vi "Dashboard Main.vi"() -> ()   [LabVIEW 2015]
uses:
  <vilib>/Utility/miscctls.llb/LVRowAndColumnTypeDef.ctl
  <vilib>/event_ctls.llb/eventvkey.ctl
  <vilib>/Rock Robotics/WPI/Dashboard/WPI_DashboardLogging Global.vi
  <vilib>/Rock Robotics/Network Tables/NT Read Numeric Array.vi
  <vilib>/Utility/config.llb/Write Key (String).vi
  <vilib>/Utility/config.llb/Write Key (I32).vi
  <vilib>/Utility/config.llb/NI_LVConfig.lvlib
  <vilib>/vision/NI_Vision_Development_Module.lvlib
panel:
  out "fps 2":dbl format="%#.1g"
  in  "Camera Settings 2":T1={"Frame Rate"=30, "Compression"=30, "Size"=1} {"Frame Rate" scale=1.0..30.0; "Size" items=["640x480", "320x240", "160x120"]}
  in  "Vision 2":u16(ring) items=["Camera Off", "USB Camera SW", "USB Camera HW", "IP Camera"]
  out "Mbps 2":dbl format="%#.1g"
  in  "TCP":refnum<k5>
  in  "Rec Mode":enum32{"Stop", "Record", "Playback"}(radio)
  in  "Vision":u16(ring) items=["Camera Off", "USB Camera SW", "USB Camera HW", "IP Camera"]
  out "Camera IP":string
  out "Image Message":string="Timeout in Camera Communications"
  in  "Dashboard Tab":T2(tab)
  in  "Select Auto":string(combo)
  out "NT Connection":bool
  in  "Camera Settings":T1={"Frame Rate"=30, "Compression"=30, "Size"=1} {"Frame Rate" scale=1.0..30.0; "Size" items=["640x480", "320x240", "160x120"]}
  out "MotorChart R":cluster{"Numeric":dbl, "Numeric":dbl}(graph)
  out "MotorChart L":T3(graph)
  out "MotorSliders R":cluster{"MotorSlide1":dbl, "MotorSlide2":dbl} {"MotorSlide2" scale=-1.0..1.0 scale format="%#_2e"; "MotorSlide1" scale=-1.0..1.0 scale format="%#_2e"}
  out "MotorSliders L":T4 {"MotorSlide4 2" scale=0.0..14.0 scale format="%#_2e"; "MotorSlide2" scale=-1.0..1.0 scale format="%#_2e"; "MotorSlide1" scale=-1.0..1.0 scale format="%#_2e"}
  out "Gyro":dbl(knob) scale=0.0..360.0
  out "JS1 Z":dbl(slide) scale=-1.0..1.0 scale format="%#_2e"
  out "JS1 Graph":cluster{"X":dbl, "Y":dbl}[](graph)
  out "JS1 Buttons":T5
  out "JS2 Z":dbl(slide) scale=-1.0..1.0 scale format="%#_2e"
  out "JS2 Graph":cluster{"X":dbl, "Y":dbl}[](graph)
  out "JS2 Buttons":T5
  out "Mode":T6(ring)=enum."Auto Disabled"
  in  "DB Camera Config":bool
  out "fps":dbl format="%#.1g"
  out "Mbps":dbl format="%#.1g"
  out "Mbps LED":bool
  in  "DB/String 9":string
  in  "DB/String 8":string
  in  "DB/String 7":string
  in  "DB/String 6":string
  in  "DB/String 5":string
  in  "DB/String 4":string
  in  "DB/String 3":string
  in  "DB/String 2":string
  in  "DB/String 1":string
  in  "DB/String 0":string
  in  "DB/Slider 0":dbl(slide) scale=0.0..5.0
  in  "DB/Slider 1":dbl(slide) scale=0.0..5.0
  in  "DB/Slider 2":dbl(slide) scale=0.0..5.0
  in  "DB/Slider 3":dbl(slide) scale=0.0..5.0
  out "DB/LED 3":bool
  out "DB/LED 2":bool
  out "DB/LED 1":bool
  out "DB/LED 0":bool
  in  "DB/Button 3":bool
  in  "DB/Button 2":bool
  in  "DB/Button 1":bool
  in  "DB/Button 0":bool caption="New Name"
  in  "Test Slider":dbl(slide) scale=0.0..100.0 scale format="%#_3g"
  in  "On/Off":bool caption="Solenoid"
  in  "Test Name":u16(ring) items=["Select the test to run..."]
  in  "Test Tree":string(tree)
  in  "Motor":cluster{"Value":dbl, "Enable":bool} {"Value" scale=-1.0..1.0 scale format="%#_3g"}
  out "Progress":T7 {"Test Progress" scale=0.0..100.0}
  in  "Rev/Fwd":cluster{"Forward":bool, "Reverse":bool}
  in  "Test Ring":u16(ring) items=["Monochrome", "Color"]
  out "Cmd Status":string
  in  "Execute Command":bool
  in  "Command Params":string[][](table)
  in  "Command Selection":i32(listbox)
  in  "CheckList":i32(listbox)
  out "Tree":string(tree)
  out "Camera Image":T8(plugin-control)
  out "Background":bool
  # "Left"
  # "Front"
  # "Right"
  # "Battery"
  # "This tab is a great place for autonomous settings and robot-specific values.\nPlace controls and indicators inside this tab and match name to\nDashboard Variables on robot. You can also delete this comment."
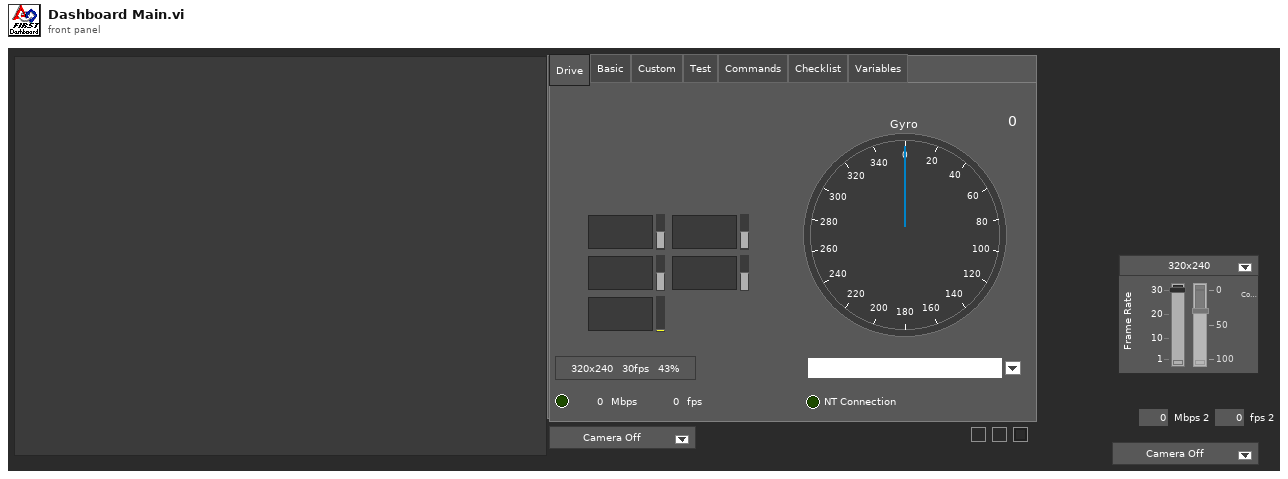
[diagram p1: front panel]
types:
  T1 = cluster{"Frame Rate":i32, "Compression":i32, "Size":u16}
  T2 = enum32{"Drive", "Basic", "Custom", "Test", "Commands", "Checklist", "Variables"}
  T3 = cluster{"Numeric":dbl, "Numeric":dbl, "Battery V":dbl}
  T4 = cluster{"MotorSlide1":dbl, "MotorSlide2":dbl, "MotorSlide4 2":dbl}
  T5 = cluster{bool, bool, bool, bool, bool, bool, bool, bool, bool, bool, bool, bool}
  T6 = enum8{"Tele-Op Disabled", "Tele-Op Enabled", "Auto Disabled", "Auto Enabled", "Test Disabled", "Test Enabled", "Disconnected", "No Code", "E-Stop"}
  T7 = cluster{"Test Progress":u8, "Test Progress Text":string}
  T8 = typedef "IMAQ Image.ctl" = refnum<image>
  T9 = typedef "Image Type" = u32
  T10 = cluster{"IDs":cluster{"RPC field ID":u16, "Unique ID":u16}, "String":string}
  T11 = enum32{"Drive", "Basic", "Custom", "Test", "Checklist", "Variables"}
  T12 = cluster{"Camera Image":refnum<vi>, "Dashboard Tab":refnum<vi>, "Background":refnum<vi>, "Vision":refnum<vi>, "Rec Mode":refnum<vi>, "Test Slider":refnum<vi>, "On/Off ":refnum<vi>, "Test Ring":refnum<vi>, "Rev/Fwd":refnum<vi>, "Test Name":refnum<vi>, "Motor":refnum<vi>, "Progress":refnum<vi>, "CheckList":refnum<vi>, "Tree":refnum<vi>, "Test Tree":refnum<vi>, "Command Params":refnum<vi>, "Command Selection":refnum<vi>, "Execute Command":refnum<vi>, "Cmd Status":refnum<vi>}
  T13 = cluster{"Error Strings":string, "Disable Counts":cluster{u16, u16}, "Rail Faults":cluster{u16, u16, u16}, "Robot IP":string, "DB Mode":u8, "Event Info":cluster{"Name":string, "Type":u8, "Number":u16, "Replay":u8}, "Camera Addr":string}
  T14 = cluster{"Storage":cluster{"Disk Free":u64, "RAM Block":u32, "RAM free":u32}, "CPU Utilization":cluster{"CPU % ISR":sgl, "CPU % Time Crit":sgl, "CPU % Timed Str":sgl, "CPU % High":sgl, "CPU % Above":sgl, "CPU % Normal":sgl, "CPU % Low":sgl}, "CAN":cluster{"% Bus Utilization":sgl, "Bus Off Cnt":u32, "TX_FIFO Full Cnt":u32, "Receive Error Cnt":u8, "Transmit Error Cnt":u8}, "HID":cluster{"HID Outputs":u32, "Rumble Low":u16, "Rumble High":u16}[]}
  T15 = cluster{"Status bits":cluster{"Test Mode":bool, "Autonomous":bool, "Enabled":bool, "Code Start":bool, "Brownout":bool, "Reserved 2":bool, "Reserved 3":bool, "E-Stop":bool}, "Code Trace":cluster{"Disabled":bool, "TeleOp":bool, "Auto":bool, "Test":bool}, "Controller Type":enum16{"unknown", "cRIO", "roboRio"}, "Code?":enum16{"unknown", "noCode", "code"}, "Battery V":dbl}
  T16 = cluster{"Control Bits":cluster{"TestMode":bool, "Autonomous":bool, "Enabled":bool, "FMS Present":bool, bool, bool, bool, "E-Stop":bool}, "Team Station ":u8, "Countdown":sgl, "Joystick Values":cluster{"Axes":dbl[], "Buttons":bool[], "POVs":i16[]}[]}
  T17 = cluster{"Axes":dbl[], "Buttons":bool[], "POVs":i16[]}[]
  T18 = cluster{"Axes":dbl[], "Buttons":bool[], "POVs":i16[]}
  T19 = cluster{"Buttons[0]":bool, "Buttons[1]":bool, "Buttons[2]":bool, "Buttons[3]":bool, "Buttons[4]":bool, "Buttons[5]":bool, "Buttons[6]":bool, "Buttons[7]":bool, "Buttons[8]":bool, "Buttons[9]":bool, "Buttons[10]":bool, "Buttons[11]":bool}
  T20 = typedef "NI_LVConfig.lvlib/Config Data RefNum.ctl" = refnum<k1>
  T21 = cluster{"Operation":enum16{"Update", "Clear"}, "Color Box":u32}[]
  T22 = typedef "eventvkey.ctl" = enum16{"ASCII", "Enter", "Return", "Shift", "Ctrl", "Alt", "Cmd", "Opt", "Caps", "NumLock", "Clear", "Break", "Up", "Down", "Left", "Right", "Insert", "Delete", "Home", "End", "PageUp", "PageDown", "Escape", "Help", "Pause", "ScrollLock", "F1", "F2", "F3", "F4", "F5", "F6", "F7", "F8", "F9", "F10", "F11", "F12", "F13", "F14", "F15", "F16", "F17", "F18", "F19", "F20", "F21", "F22", "F23", "F24", "Play", "VolumeUp", "VolumeDown", "Mute", "Two Byte Char"}
  T23 = cluster{"Image Size":bool, "Image Type":bool, "Pixel Value":bool, "ROI Information":bool, "Zoom Factor":bool}
  T24 = enum8{"Enabled", "Disabled", "Disabled and Grayed Out"}
  T25 = cluster{"Operation":enum16{"Update", "Clear"}, "Color Box":u32}
  T26 = typedef "LVRowAndColumnTypeDef.ctl" = cluster{"Row":i32, "Column":i32}
  T27 = cluster{"Shift":bool, "Ctrl":bool, "Alt":bool, "Cmd":bool, "Opt":bool}
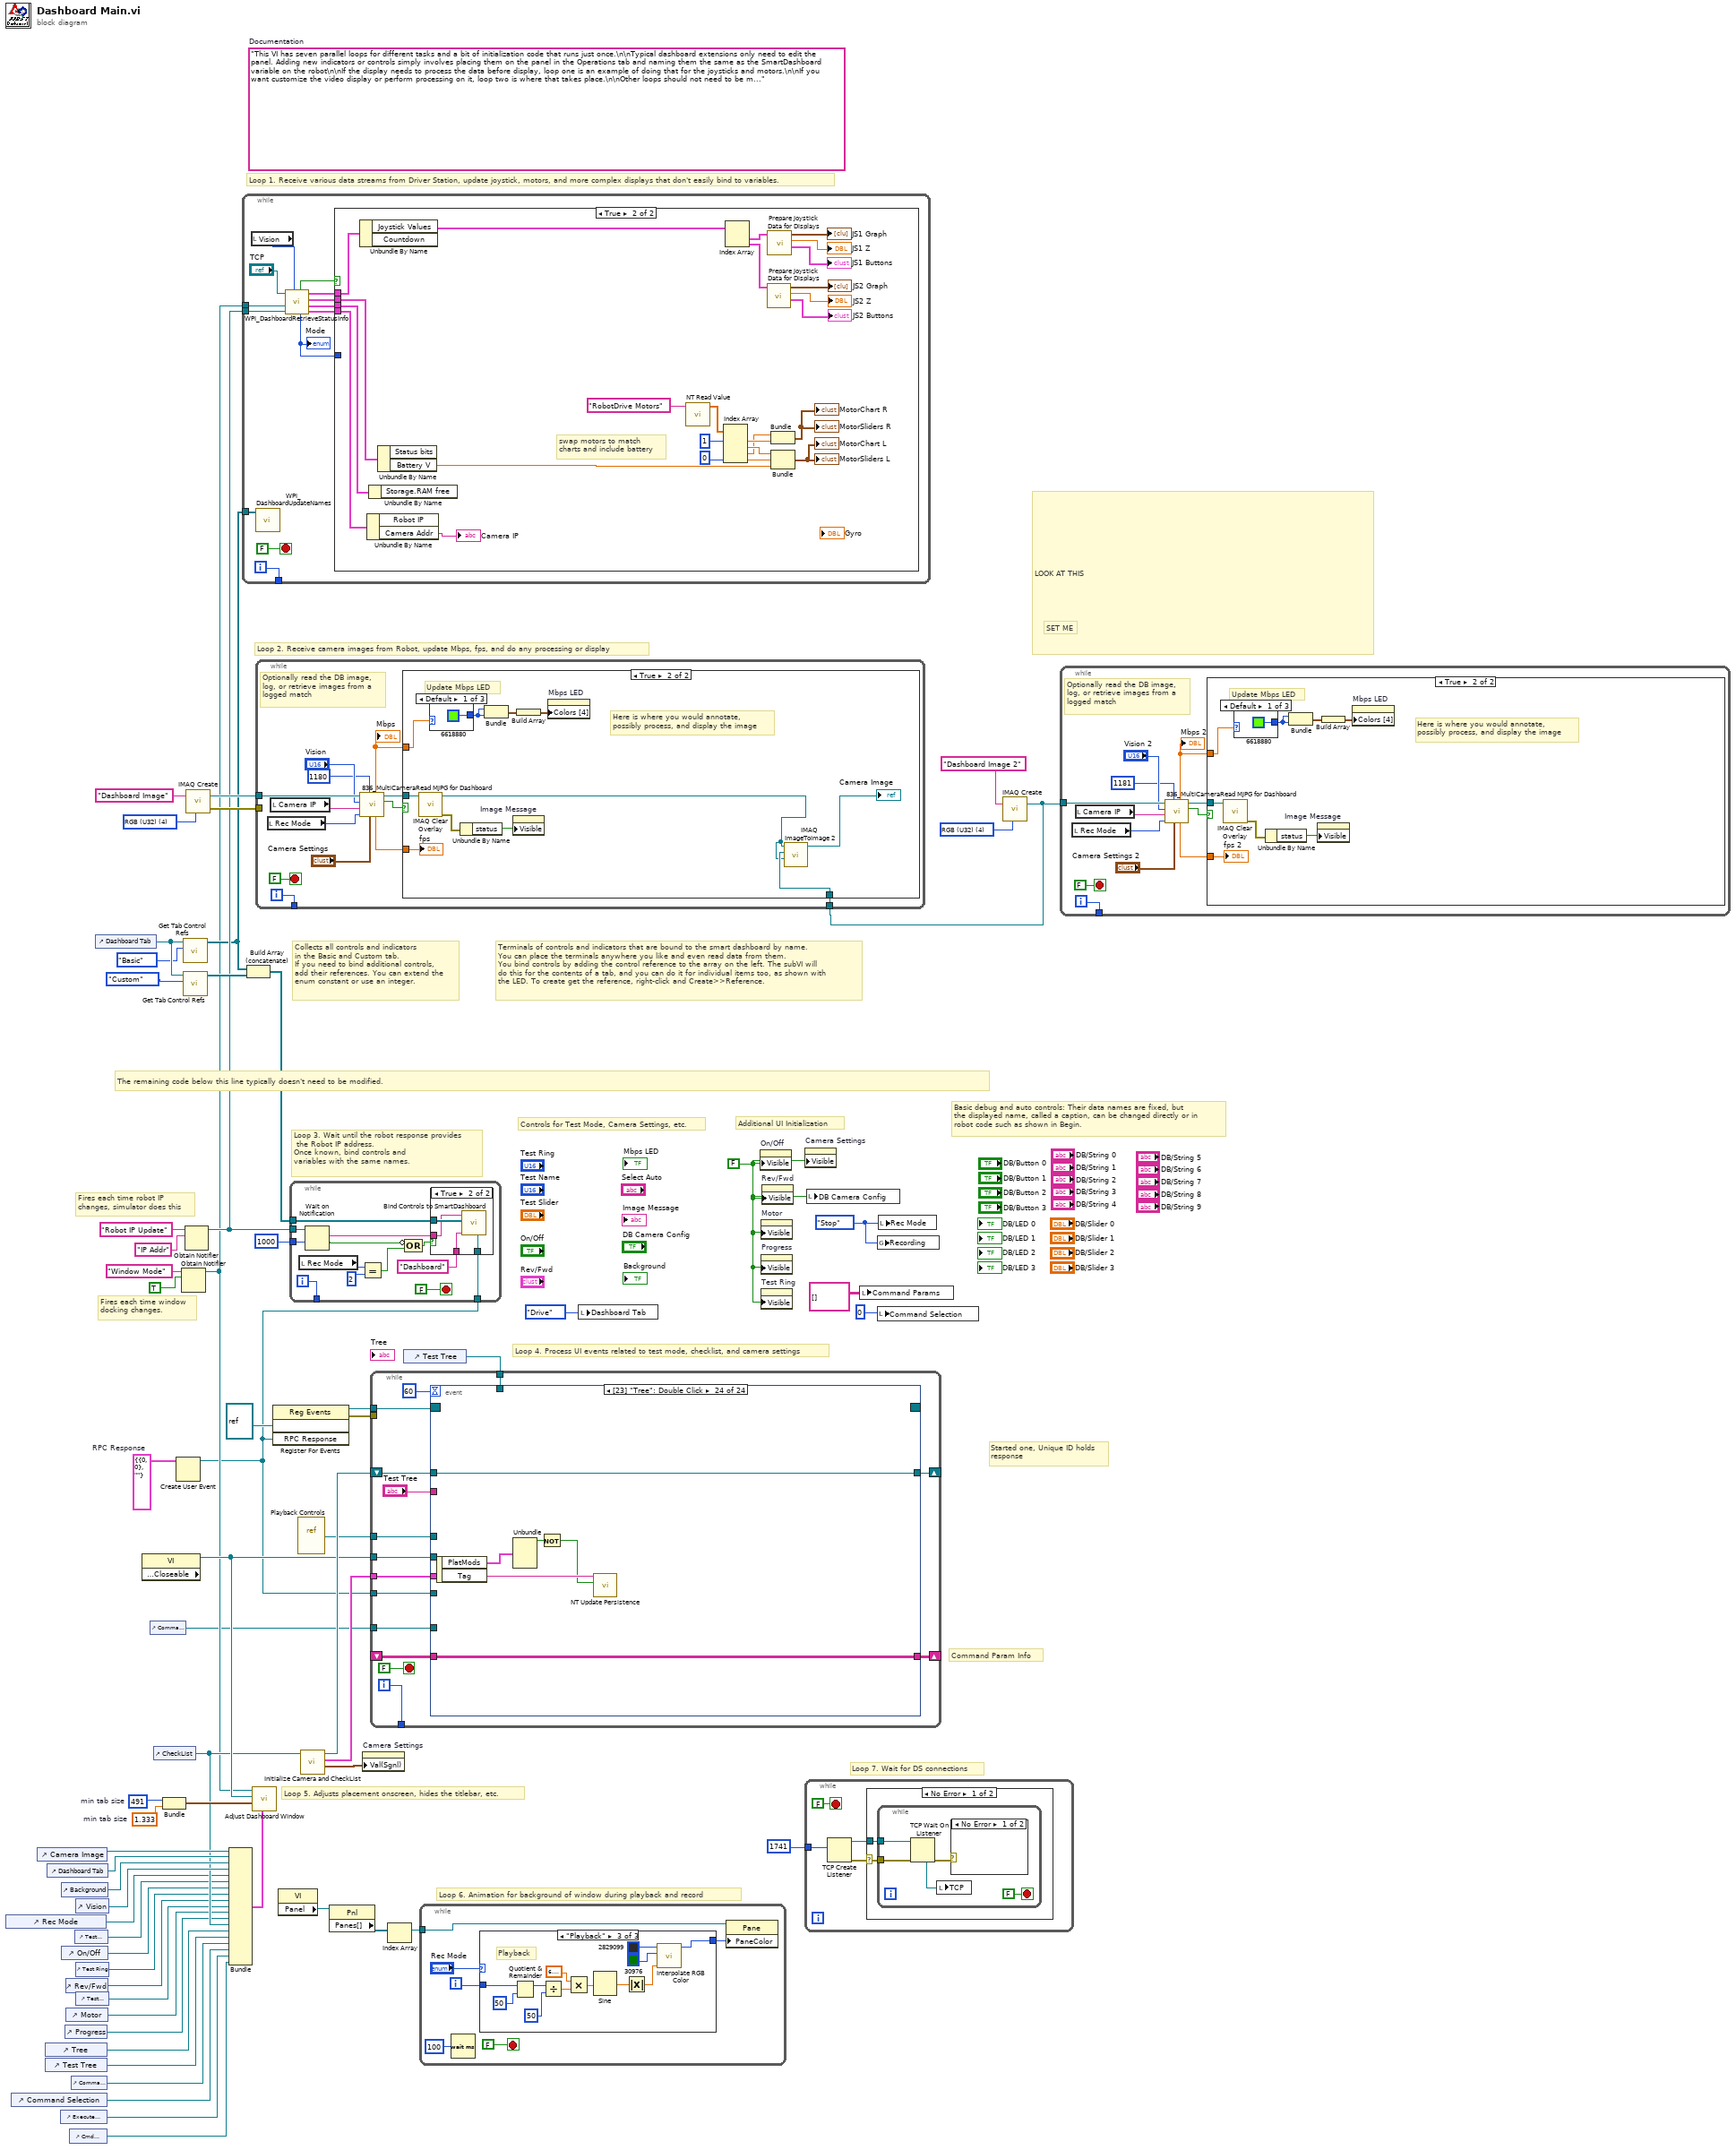
[diagram p0: block diagram]
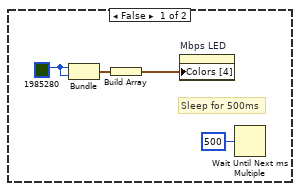
[diagram p2: hidden frame]
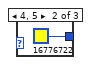
[diagram p3: hidden frame]
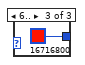
[diagram p4: hidden frame]
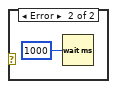
[diagram p5: hidden frame]
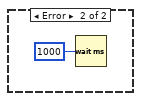
[diagram p6: hidden frame]
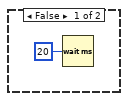
[diagram p7: hidden frame]
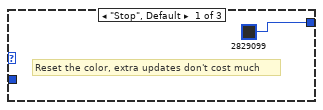
[diagram p8: hidden frame]
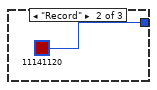
[diagram p9: hidden frame]
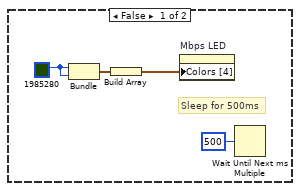
[diagram p11: hidden frame]
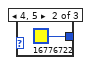
[diagram p12: hidden frame]
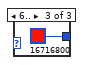
[diagram p13: hidden frame]
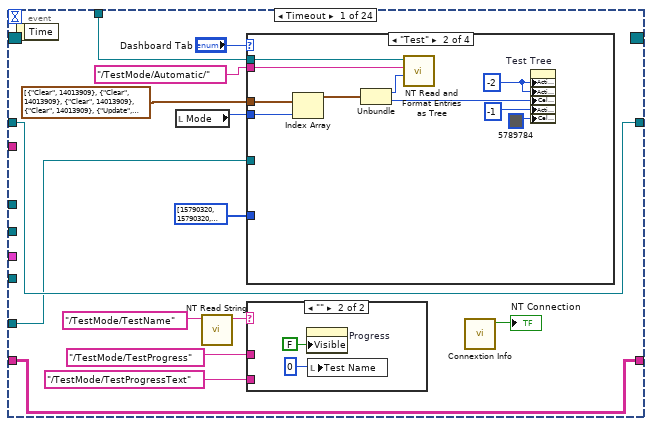
[diagram p14: hidden frame]
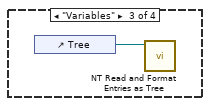
[diagram p16: hidden frame]
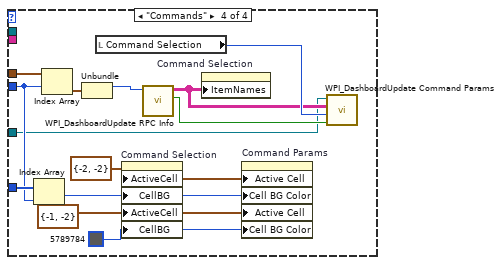
[diagram p17: hidden frame]
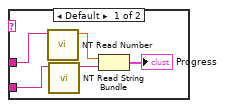
[diagram p18: hidden frame]
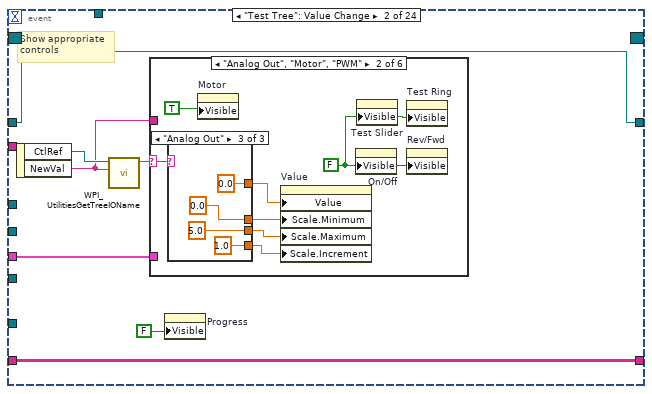
[diagram p19: hidden frame]
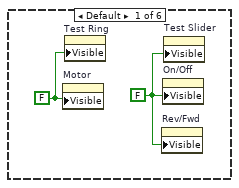
[diagram p20: hidden frame]
diagram:
  w2 = T9 4 items=["Grayscale (U8)", "Grayscale (I16)", "Grayscale (SGL)", "Complex (CSG)", "RGB (U32)", "HSL (U32)", "RGB (U64)"] ("Image Type")
  w10 = T10 {"IDs"={"RPC field ID"=0, "Unique ID"=0}, "String"=""}  # RPC Response
  w36 = 491  # min tab size
  w35 = 1.333  # min tab size
  w44 = enum32{"Stop", "Record", "Playback"}."Stop" ("Rec Mode")
  w18 = FALSE ("Visible")
  (unwired) "This VI has seven parallel loops for different tasks and a bit of initialization code that runs just once.\n\nTypical dashboard extensions only need to edit the panel. Adding new indicators or controls simply involves placing them on the panel in the Operations tab and naming them the same as the SmartDashboard variable on the robot\n\nIf the display needs to process the data before display, loop one is an example of doing that for the joysticks and motors.\n\nIf you want customize the video display or perform processing on it, loop two is where that takes place.\n\nOther loops should not need to be modified. They are pretty standard, and document the task they perform."  # Documentation
  w64 = T9 4 items=["Grayscale (U8)", "Grayscale (I16)", "Grayscale (SGL)", "Complex (CSG)", "RGB (U32)", "HSL (U32)", "RGB (U64)"] ("Image Type")
  # "SET ME"
  # "LOOK AT THIS"
  # "Command Param Info"
  # "Started one, Unique ID holds\nresponse"
  # "Loop 7. Wait for DS connections"
  # "Basic debug and auto controls: Their data names are fixed, but\nthe displayed name, called a caption, can be changed directly or in\nrobot code such as shown in Begin."
  # "Controls for Test Mode, Camera Settings, etc."
  # "Additional UI Initialization"
  # "Loop 6. Animation for background of window during playback and record"
  # "Fires each time robot IP\nchanges, simulator does this"
  # "Fires each time window\ndocking changes."
  # "Collects all controls and indicators\nin the Basic and Custom tab.\nIf you need to bind additional controls,\nadd their references. You can extend the\nenum constant or use an integer."
  # "The remaining code below this line typically doesn't need to be modified."
  # "Loop 4. Process UI events related to test mode, checklist, and camera settings"
  # "Terminals of controls and indicators that are bound to the smart dashboard by name.\nYou can place the terminals anywhere you like and even read data from them.\nYou bind controls by adding the control reference to the array on the left. The subVI will\ndo this for the contents of a tab, and you can do it for individual items too, as shown with\nthe LED. To create get the reference, right-click and Create>>Reference."
  # "Loop 3. Wait until the robot response provides\n the Robot IP address.\nOnce known, bind controls and\nvariables with the same names."
  # "Loop 5. Adjusts placement onscreen, hides the titlebar, etc."
  # "Loop 1. Receive various data streams from Driver Station, update joystick, motors, and more complex displays that don't easily bind to variables."
  # "Loop 2. Receive camera images from Robot, update Mbps, fps, and do any processing or display"
  n1 = control-ref of="Rec Mode"() -> (w24:refnum<vi>)
  n2 = control-ref of="Command Selection"() -> (w9:refnum<vi>)
  n3 = control-ref of="Camera Image"() -> (w39:refnum<vi>)
  n4 = control-ref of="Tree"() -> (w28:refnum<vi>)
  n5 = control-ref of="Test Tree"() -> (w27:refnum<vi>)
  n6 = control-ref of="Dashboard Tab"() -> (w38:refnum<vi>)
  n7 = control-ref of="Execute Command"() -> (w11:refnum<vi>)
  n8 = control-ref of="Background"() -> (w33:refnum<vi>)
  n9 = control-ref of="On/Off"() -> (w22:refnum<vi>)
  n10 = control-ref of="Progress"() -> (w19:refnum<vi>)
  n11 = control-ref of="Rev/Fwd"() -> (w20:refnum<vi>)
  n12 = control-ref of="Motor"() -> (w25:refnum<vi>)
  n13 = control-ref of="Cmd Status"() -> (w5:refnum<vi>)
  n14 = control-ref of="Command Params"() -> (w12:refnum<vi>)
  n15 = control-ref of="Test Slider"() -> (w23:refnum<vi>)
  n16 = control-ref of="Vision"() -> (w37:refnum<vi>)
  n17 = control-ref of="Test Ring"() -> (w21:refnum<vi>)
  n18 = control-ref of="Test Name"() -> (w26:refnum<vi>)
  n19 = control-ref of="Dashboard Tab"() -> (w42:refnum<vi>)
  n20 = property class="VI" props=["Front Panel.Closeable"]() -> (reference out=w43:refnum<vi>)  [unwired: 2 in, 2 out]
  n21 = control-ref of="Command Params"() -> (w4:refnum<vi>)
  n22 = control-ref of="CheckList"() -> (w29:refnum<vi>)
  n23 = Bundle("min tab size"=w36, "min tab size"=w35) -> (w34:cluster{"min tab size":i32, "min tab size":dbl})  [unwired: 1 in]
  n24 = Create User Event(user event datatype=w10) -> (user event=w6:refnum<user-event>)  [unwired: 1 in, 1 out]
  n25 = Obtain Notifier(name (unnamed)="Window Mode", notification data type=TRUE) -> (notifier out=w15:refnum<notifier>)  [unwired: 2 in, 2 out]
  n26 = call <vilib>:"Get Tab Control Refs.vi"("Page Index"=T11."Basic" ("Dashboard Tab"), "TabControl in"=w42) -> ("ControlsOnPage"=w16:refnum<vi>[])  [unwired: 9 in]
  n27 = call <vilib>:"Get Tab Control Refs.vi"("Page Index"=T11."Custom" ("Dashboard Tab"), "TabControl in"=w42) -> ("ControlsOnPage"=w41:refnum<vi>[])  [unwired: 9 in]
  n28 = Obtain Notifier(name (unnamed)="Robot IP Update", notification data type="IP Addr" ("name (unnamed)")) -> (notifier out=w17:refnum<notifier>)  [unwired: 2 in, 2 out]
  n29 = call "IMAQ Create"("Image Name"="Dashboard Image", "Image Type"=w64) -> ("New Image"=w62:T8, "error out"=w61:errorcluster)  [unwired: 2 in, 1 out]
  n30 = Bundle("Camera Image"=w39, "Dashboard Tab"=w38, "Background"=w33, "Vision"=w37, "Rec Mode"=w24, "Test Slider"=w23, "On/Off"=w22, "Test Ring"=w21, "Rev/Fwd"=w20, "Test Name"=w26, "Motor"=w25, "Progress"=w19, "CheckList"=w29, "Tree"=w28, "Test Tree"=w27, "Command Params"=w12, "Command Selection"=w9, "Execute Command"=w11, "Cmd Status"=w5) -> (w30:T12)  [unwired: 1 in]
  n31 = while {
    tunnel: [w76] -> _
    tunnel: w17 -> [w70]
    tunnel: w16 -> [w69]
    tunnel: w15 -> [w65]
    i -> [w76]
    stop <- FALSE stop-if-true
    n32 = local read "Vision"() -> (w67:u16)
    n33 = call <vilib>:"WPI_DashboardUpdateNames.vi"("Controls on Tab"=w69) -> ()  [unwired: 11 in]
    n34 = call <vilib>:"WPI_DashboardRetrieveStatusInfo.vi"("Vision"=w67, "Binding Refnum"=w70, "Window Mode Notifier"=w65, "TCP Cnx"="TCP") -> ("Power and Errors"=w71:T13, "Robot Metrics"=w74:T14, "Status Info"=w75:T15, "Control Info"=w72:T16, "Robot Mode"=w68:T6, "Process?"=w73:bool)  [unwired: 2 in]
    "Mode" <- w68
    n35 = case shown="True" w73 {
      tunnel: w75 -> [_ w103]
      tunnel: w74 -> [_ w102]
      tunnel: w72 -> [_ w101]
      tunnel: w71 -> [_ w100]
      tunnel: w68 -> [_ _]
      frame False {
        n36 = Wait (ms)(milliseconds to wait=u32 20) -> ()  [unwired: 1 out]
      }
      frame True {
        # "swap motors to match\ncharts and include battery"
        n37 = Unbundle By Name(w101) -> ("Joystick Values"=w90:T17)  [unwired: 1 out]
        n38 = Unbundle By Name(w100) -> ("Camera Addr"=→"Camera IP":string)  [unwired: 1 out]
        n39 = Unbundle By Name(w102) -> ()  [unwired: 1 out]
        n40 = Unbundle By Name(w103) -> ("Battery V"=w91:dbl)  [unwired: 1 out]
        n41 = call-poly <vilib>:"NT Read Value.vi"("Name"="RobotDrive Motors") -> ("Numeric Array"=w79:dbl[])  [unwired: 9 in, 1 out]
        n42 = Index Array(array=w79, index #1=1, index #4=0) -> (element #1=w95:dbl, element #2=w96:dbl, element #3=w94:dbl, element #4=w99:dbl)  [unwired: 2 in]
        n43 = Index Array(array=w90) -> (element #1=w89:T18, element #2=w84:T18)  [unwired: 2 in]
        n44 = call "Prepare Joystick Data for Displays.vi"("Joystick Values"=w84) -> ("Buttons"=→"JS2 Buttons":T19, "Z Axis"=→"JS2 Z":dbl, "Cartesian Data"=→"JS2 Graph":cluster{"X axis":dbl, "X axis":dbl}[])  [unwired: 8 in]
        n45 = call "Prepare Joystick Data for Displays.vi"("Joystick Values"=w89) -> ("Buttons"=→"JS1 Buttons":T19, "Z Axis"=→"JS1 Z":dbl, "Cartesian Data"=→"JS1 Graph":cluster{"X axis":dbl, "X axis":dbl}[])  [unwired: 8 in]
        n46 = Bundle("Numeric"=w94, "Numeric"=w95) -> (→"MotorChart R" →"MotorSliders R":cluster{"Numeric":dbl, "Numeric":dbl})  [unwired: 1 in]
        n47 = Bundle("Numeric"=w96, "Numeric"=w99, "Battery V"=w91) -> (→"MotorChart L" →"MotorSliders L":T3)  [unwired: 1 in]
      }
    }
  }
  n48 = Build Array (concatenate)(w16, w41) -> (w40:refnum<vi>[])
  n49 = call "Adjust Dashboard Window.vi"("Sizing Refnums"=w30, "Size Constraints"=w34, "VI"=w43, "WIn Mode"=w15) -> ()  [unwired: 8 in]
  n50 = register-events(refnum<vi> refnum, w6) -> (reference out=w48:refnum<event-registration>, error out=w47:errorcluster)  [unwired: 2 in]
  n51 = property class="VI"() -> ("Panel"=w51:refnum<vi>)  [unwired: 2 in, 2 out]
  n52 = while {
    tunnel: w40 -> [w116]
    tunnel: w17 -> [w114]
    tunnel: [w112] -> _
    tunnel: u32 1000 ("milliseconds to wait") -> [w111]
    tunnel: w6 -> [w104]
    i -> [w112]
    stop <- FALSE stop-if-true
    n53 = local read "Rec Mode"() -> (w107:enum32{"Stop", "Record", "Playback"})
    n54 = Wait on Notification(notifier=w114, timeout in ms (-1)=w111) -> (notification=w113:string, timed out?=w109:bool)  [unwired: 2 in, 2 out]
    n55 = Equal?(x=w107, y=u16 2 ("Rec Mode")) -> (x = y?=w108:bool)
    n56 = Compound Arithmetic op=OR(invert w109, w108) -> (w110:bool)
    n57 = case shown="True" w110 {
      tunnel: w116 -> [_ w120]
      tunnel: w113 -> [_ w119]
      tunnel: "Dashboard" -> [_ w118]
      tunnel: w104 -> [_ w117]
      frame False {
      }
      frame True {
        n58 = call <vilib>:"Bind Controls to SmartDashboard.vi"("RPC ref"=w117, "Client Name"=w118, "Bound Control Refs"=w120, "Server IP Address"=w119) -> ()  [unwired: 8 in]
      }
    }
  }
  n59 = vi-ref "Playback Controls.vi"() -> (w49:refnum<vi>)
  n60 = call "Initialize Camera and CheckList.vi"("ListBox in"=w29) -> ("Cluster"=w55:cluster{"value":i32, "value":i32, "index":i32}, "Array"=w56:cluster{string[]}[], "File Refnum"=w54:T20)  [unwired: 8 in]
  n61 = property class="Pnl"(reference=w51) -> ("Panes[]"=w52:refnum<vi>[])  [unwired: 1 in, 2 out]
  n62 = property on="Camera Settings" class="Clust (strict)"("Val(Sgnl)"=w55) -> ()  [unwired: 2 in, 2 out]
  n63 = Index Array(array=w52) -> (element=w50:refnum<vi>)  [unwired: 1 in]
  n64 = control-ref of="Test Tree"() -> (w53:refnum<vi>)
  n65 = while {
    tunnel: w56 -> [w132]
    shift-right: [w131] -> _
    shift-left: w54 -> [w130]
    tunnel: [w129] -> _
    tunnel: w53 -> [w128]
    tunnel: w49 -> [w127]
    tunnel: w48 -> [w126]
    tunnel: w47 -> [_]
    tunnel: w43 -> [w125]
    tunnel: w6 -> [w124]
    tunnel: w4 -> [w123]
    shift-right: [w122] -> _
    shift-left: _ -> [w121]
    i -> [w129]
    stop <- FALSE stop-if-true
    n66 = event shown="[23] \"Tree\": Double Click" {
      selector: w126 -> [_ _ _ _ _ _ _ _ _ _ _ _ _ _ _ _ _ _ _ _ _ _ _ _]
      dyn-events: [_ _ _ _ _ _ _ _ _ _ _ _ _ _ _ _ _ _ w441 _ _ _ _ _] -> _
      timeout: u32 60 ("milliseconds to wait") -> [_ _ _ _ _ _ _ _ _ _ _ _ _ _ _ _ _ _ _ _ _ _ _ _]
      tunnel: w128 -> [w145 _ _ _ _ _ _ _ _ _ _ _ _ _ _ _ _ _ _ _ _ _ _ _]
      tunnel: "Test Tree" -> [_ _ _ _ _ _ _ _ _ _ _ _ _ w404 w413 w416 w421 w430 _ _ _ _ _ _]
      tunnel: w132 -> [_ w183 _ _ _ _ _ _ _ _ _ w366 w397 _ _ _ _ _ _ _ _ _ _ _]
      tunnel: [w142 w182 w286 w292 w302 w306 w312 w324 w332 w338 w351 w365 w390 w403 w411 w415 w420 w429 w443 w459 w461 w469 w480 w485] -> w131
      tunnel: w130 -> [w142 w182 w286 w292 w302 w306 w312 w324 w332 w338 w351 w364 w390 w403 w411 w415 w420 w429 w443 w459 w461 w469 w480 w485]
      tunnel: w127 -> [_ _ _ _ _ _ _ _ _ _ _ _ _ _ _ _ _ _ w444 _ w464 _ _ _]
      tunnel: w125 -> [_ _ _ _ _ _ _ _ _ _ _ _ _ _ _ _ _ _ w439 _ _ _ _ _]
      tunnel: w124 -> [_ _ _ _ _ _ _ _ _ _ _ _ _ _ _ _ _ _ w435 _ _ _ _ _]
      tunnel: w123 -> [w137 _ _ _ _ _ w310 _ _ _ _ _ _ _ _ _ _ _ _ _ _ _ _ _]
      tunnel: [w136 w181 w285 w291 w301 w307 w308 w318 w329 w337 w350 w363 w389 w402 w410 w414 w419 w428 w434 w457 w460 w465 w473 w486] -> w122
      tunnel: w121 -> [w136 w181 w285 w291 w301 w307 w308 _ _ w337 w350 w363 w389 w402 w410 w414 w419 w428 w434 w457 w460 w465 w473 w486]
      event Timeout {
        n67 = event-data() -> ()  [unwired: 1 in, 1 out]
        n68 = local read "Mode"() -> (w139:T6)
        n69 = call <vilib>:"NT Read String.vi"("Name"="/TestMode/TestName") -> ("String"=w148:string)  [unwired: 9 in, 1 out]
        n70 = case shown="\"Test\"" "Dashboard Tab" {
          tunnel: w145 -> [_ w159 _ _]
          tunnel: "/TestMode/Automatic/" ("Name Pattern") -> [_ w158 _ _]
          tunnel: T21 [{"Operation"=enum."Clear", "Color Box"=14013909}, {"Operation"=enum."Clear", "Color Box"=14013909}, {"Operation"=enum."Clear", "Color Box"=14013909}, {"Operation"=enum."Clear", "Color Box"=14013909}, {"Operation"=enum."Update", "Color Box"=14013909}, {"Operation"=enum."Update", "Color Box"=16777215}, {"Operation"=enum."Clear", "Color Box"=14013909}, {"Operation"=enum."Clear", "Color Box"=14013909}, {"Operation"=enum."Clear", "Color Box"=14013909}] -> [_ w151 _ w168]
          tunnel: w139 -> [_ w150 _ w167]
          tunnel: u32[] [15790320, 15790320, 15790320, 15790320, 16777215, 16777215, 15790320, 15790320, 15790320] -> [_ _ _ w173]
          tunnel: w137 -> [_ _ _ w161]
          frame "Custom", Default {
          }
          frame "Test" {
            w157 = -2 ("Active Item:Row Number")
            n71 = Index Array(array=w151, index=w150) -> (element=w152:T25)
            n72 = Unbundle(w152) -> ("Operation"=w153:enum16{"Update", "Clear"}, "Color Box"=w154:u32)
            n73 = call <vilib>:"NT Read and Format Entries as Tree.vi"("Operation"=w153, "Name Pattern"=w158, "Tree Refnum"=w159) -> ()  [unwired: 7 in, 2 out]
            n74 = property on="Test Tree" class="Tree (strict)"("Active Item Row Number"=w157, "ActiveColNum"=w157, "CellBG"=w154, "Active Item Row Number"=-1 ("Active Item:Row Number"), "CellBG"=u32 5789784 ("Color Box")) -> ()  [unwired: 2 in, 2 out]
          }
          frame "Variables" {
            n75 = control-ref of="Tree"() -> (w160:refnum<vi>)
            n76 = call <vilib>:"NT Read and Format Entries as Tree.vi"("Tree Refnum"=w160) -> ()  [unwired: 9 in, 2 out]
          }
          frame "Commands" {
            w169 = u32 5789784 ("Color Box")
            w170 = T26 {"Row"=-1, "Column"=-2} ("Active Cell:Active Cell")
            w172 = T26 {"Row"=-2, "Column"=-2} ("Active Cell:Active Cell")
            n77 = Index Array(array=w173, index=w167) -> (element=w171:u32)
            n78 = Index Array(array=w168, index=w167) -> (element=w166:T25)
            n79 = Unbundle(w166) -> ("Operation"=w165:enum16{"Update", "Clear"})  [unwired: 1 out]
            n80 = local read "Command Selection"() -> (w164:i32)
            n81 = property on="Command Selection" class="MCListbox (strict)"("ActiveCell"=w172, "CellBG"=w171, "ActiveCell"=w170, "CellBG"=w169) -> ()  [unwired: 2 in, 2 out]
            n82 = call <vilib>:"WPI_DashboardUpdate RPC Info.vi"("Operation"=w165) -> ("update"=w163:bool, "commands"=w162:string[][])  [unwired: 9 in]
            n83 = property on="Command Selection" class="MCListbox (strict)"("ItemNames"=w162) -> ()  [unwired: 2 in, 2 out]
            n84 = property on="Command Params" class="Tbl (strict)"("Active Cell"=w172, "Cell BG Color"=w171, "Active Cell"=w170, "Cell BG Color"=w169) -> ()  [unwired: 2 in, 2 out]
            n85 = call <vilib>:"WPI_DashboardUpdate Command Params.vi"("Update"=w163, "NewVal"=w164, "Commands"=w162, "Param Tbl"=w161) -> ()  [unwired: 7 in, 1 out]
          }
        }
        n86 = case shown="\"\"" w148 {
          tunnel: "/TestMode/TestProgress" ("Name") -> [w175 _]
          tunnel: "/TestMode/TestProgressText" ("Name") -> [w174 _]
          frame Default {
            n87 = call <vilib>:"NT Read Number.vi"("Name"=w175) -> ("Numeric"=w176:dbl)  [unwired: 9 in, 1 out]
            n88 = call <vilib>:"NT Read String.vi"("Name"=w174) -> ("String"=w177:string)  [unwired: 9 in, 1 out]
            n89 = Bundle("Numeric"=w176, "String"=w177) -> (→"Progress":cluster{"Numeric":dbl, "String":string})  [unwired: 1 in]
          }
          frame "" {
            n90 = property on="Progress" class="Clust (strict)"("Visible"=FALSE) -> ()  [unwired: 2 in, 2 out]
            n91 = local write "Test Name"(u16 0) -> ()
          }
        }
        n92 = call <vilib>:"Connextion Info.vi"() -> ("Connected"=→"NT Connection":bool)  [unwired: 10 in, 1 out]
      }
      event "Test Tree": Value Change {
        # "Show appropriate\ncontrols"
        n93 = event-data() -> ("CtlRef"=w186:refnum<vi>, "NewVal"=w184:string)  [unwired: 1 in]
        n94 = call <vilib>:"WPI_UtilitiesGetTreeIOName.vi"("NewVal"=w184, "TreeControl in"=w186) -> ("I/O Name"=w187:string)  [unwired: 9 in]
        n95 = case shown="\"Analog Out\", \"Motor\", \"PWM\"" w187 {
          selector: w187 -> [_ w194 _ w216 w225 _]
          tunnel: w184 -> [_ _ w213 w215 _ w232]
          tunnel: w183 -> [_ _ _ _ _ w231]
          frame Default {
            w189 = FALSE ("Visible")
            w188 = FALSE ("Visible")
            n96 = property on="Motor" class="Clust (strict)"("Visible"=w188) -> ()  [unwired: 2 in, 2 out]
            n97 = property on="Test Ring" class="Ring (strict)"("Visible"=w188) -> ()  [unwired: 2 in, 2 out]
            n98 = property on="Rev/Fwd" class="Clust (strict)"("Visible"=w189) -> ()  [unwired: 2 in, 2 out]
            n99 = property on="On/Off" class="Bool (strict)"("Visible"=w189) -> ()  [unwired: 2 in, 2 out]
            n100 = property on="Test Slider" class="Slide (strict)"("Visible"=w189) -> ()  [unwired: 2 in, 2 out]
          }
          frame "Analog Out", "Motor", "PWM" {
            w195 = FALSE ("Visible")
            n101 = case shown="\"Analog Out\"" w194 {
              tunnel: [1.0 ("Value") -1.0 ("Value") 0.0 ("Value")] -> w193
              tunnel: [255.0 ("Value") 1.0 ("Value") 5.0 ("Value")] -> w192
              tunnel: [128.0 ("Value") 0.0 ("Value") 0.0 ("Value")] -> w191
              tunnel: [64.0 ("Value") 0.5 ("Value") 1.0 ("Value")] -> w190
              frame "PWM" {
              }
              frame "Motor", Default {
              }
              frame "Analog Out" {
              }
            }
            n102 = property on="Motor" class="Clust (strict)"("Visible"=TRUE) -> ()  [unwired: 2 in, 2 out]
            n103 = property on="Value" class="Slide (strict)"("Value"=w191, "Scale.Minimum"=w193, "Scale.Maximum"=w192, "Scale.Increment"=w190) -> ()  [unwired: 2 in, 2 out]
            n104 = property on="On/Off" class="Bool (strict)"("Visible"=w195) -> ()  [unwired: 2 in, 2 out]
            n105 = property on="Test Slider" class="Slide (strict)"("Visible"=w195) -> ()  [unwired: 2 in, 2 out]
            n106 = property on="Test Ring" class="Ring (strict)"("Visible"=w195) -> ()  [unwired: 2 in, 2 out]
            n107 = property on="Rev/Fwd" class="Clust (strict)"("Visible"=w195) -> ()  [unwired: 2 in, 2 out]
          }
          frame "Servo" {
            w211 = FALSE ("Visible")
            n108 = call <vilib>:"NT Read Number.vi"("Name"=w213) -> ("Numeric"=w212:dbl)  [unwired: 9 in, 1 out]
            n109 = property on="Test Slider" class="Slide (strict)"("Visible"=TRUE, "Scale.Maximum"=170.0 ("Scale.Range:Maximum")) -> ()  [unwired: 2 in, 2 out]
            n110 = local write "Test Slider"(w212) -> ()
            n111 = property on="Motor" class="Clust (strict)"("Visible"=w211) -> ()  [unwired: 2 in, 2 out]
            n112 = property on="Rev/Fwd" class="Clust (strict)"("Visible"=w211) -> ()  [unwired: 2 in, 2 out]
            n113 = property on="On/Off" class="Bool (strict)"("Visible"=w211) -> ()  [unwired: 2 in, 2 out]
            n114 = property on="Test Ring" class="Ring (strict)"("Visible"=w211) -> ()  [unwired: 2 in, 2 out]
          }
          frame "Relay", "Solenoid" {
            w214 = FALSE ("Visible")
            n115 = property on="Motor" class="Clust (strict)"("Visible"=w214) -> ()  [unwired: 2 in, 2 out]
            n116 = property on="Test Slider" class="Slide (strict)"("Visible"=w214) -> ()  [unwired: 2 in, 2 out]
            n117 = Search and Replace String(input string=w215, search string="/Value  **", replace string="/Direction") -> (result string=w221:string)  [unwired: 5 in, 3 out]
            n118 = property on="Test Ring" class="Ring (strict)"("Visible"=w214) -> ()  [unwired: 2 in, 2 out]
            n119 = call <vilib>:"NT Read String.vi"("Name"=w221) -> ("String"=w219:string)  [unwired: 9 in, 1 out]
            n120 = Equal?(x="Both directions", y=w219) -> (x = y?=w217:bool)
            n121 = Not(x=w217) -> (.not. x?=w218:bool)
            n122 = property on="Rev/Fwd" class="Clust (strict)"("Visible"=w217) -> ()  [unwired: 2 in, 2 out]
            n123 = property on="On/Off" class="Bool (strict)"("Visible"=w218, "Caption.Text"=w216) -> ()  [unwired: 2 in, 2 out]
          }
          frame "Compressor", "Digital Out" {
            w224 = FALSE ("Visible")
            # "Get direction and finish"
            n124 = property on="Motor" class="Clust (strict)"("Visible"=w224) -> ()  [unwired: 2 in, 2 out]
            n125 = property on="Test Slider" class="Slide (strict)"("Visible"=w224) -> ()  [unwired: 2 in, 2 out]
            n126 = property on="Test Ring" class="Ring (strict)"("Visible"=w224) -> ()  [unwired: 2 in, 2 out]
            n127 = property on="On/Off" class="Bool (strict)"("Visible"=TRUE, "Caption.Text"=w225) -> ()  [unwired: 2 in, 2 out]
            n128 = property on="Rev/Fwd" class="Clust (strict)"("Visible"=FALSE) -> ()  [unwired: 2 in, 2 out]
          }
          frame "Camera" {
            n129 = call <vilib>:"Get Last Path Segment.vi"("String in"=w232) -> ("String out"=w233:string)  [unwired: 10 in]
            n130 = property on="On/Off" class="Bool (strict)"("Visible"=FALSE) -> ()  [unwired: 2 in, 2 out]
            n131 = property on="Motor" class="Clust (strict)"("Visible"=FALSE) -> ()  [unwired: 2 in, 2 out]
            n132 = property on="Rev/Fwd" class="Clust (strict)"("Visible"=FALSE) -> ()  [unwired: 2 in, 2 out]
            n133 = case shown="\"White Balance  **\"" w233 {
              tunnel: w232 -> [w239 w248 w257 w266 w275 _ w281]
              tunnel: w231 -> [w237 w245 w254 w263 w272 _ _]
              frame "Size  **" {
                n134 = Index Array(array=w237) -> (element=w236:cluster{string[]})  [unwired: 1 in]
                n135 = call <vilib>:"NT Read String.vi"("Name"=w239) -> ("String"=w238:string)  [unwired: 9 in, 1 out]
                n136 = Unbundle(w236) -> (w234:string[])
                n137 = Match First String(2:w234, 3:w238) -> (0:w235:i32)  [unwired: 1 out]
                n138 = property on="Test Ring" class="Ring (strict)"("Value"=w235, "Strings []"=w234) -> ()  [unwired: 2 in, 2 out]
                n139 = property on="Test Ring" class="Ring (strict)"("Visible"=TRUE) -> ()  [unwired: 2 in, 2 out]
                n140 = property on="Test Slider" class="Slide (strict)"("Visible"=FALSE) -> ()  [unwired: 2 in, 2 out]
              }
              frame "White Balance  **" {
                n141 = Index Array(array=w245, index=1) -> (element=w246:cluster{string[]})
                n142 = call <vilib>:"NT Read String.vi"("Name"=w248) -> ("String"=w247:string)  [unwired: 9 in, 1 out]
                n143 = Unbundle(w246) -> (w243:string[])
                n144 = Match First String(2:w243, 3:w247) -> (0:w242:i32)  [unwired: 1 out]
                n145 = property on="Test Ring" class="Ring (strict)"("Value"=w242, "Strings []"=w243) -> ()  [unwired: 2 in, 2 out]
                n146 = property on="Test Ring" class="Ring (strict)"("Visible"=TRUE) -> ()  [unwired: 2 in, 2 out]
                n147 = property on="Test Slider" class="Slide (strict)"("Visible"=FALSE) -> ()  [unwired: 2 in, 2 out]
              }
              frame "Exposure  **" {
                n148 = Index Array(array=w254, index=2) -> (element=w255:cluster{string[]})
                n149 = call <vilib>:"NT Read String.vi"("Name"=w257) -> ("String"=w256:string)  [unwired: 9 in, 1 out]
                n150 = Unbundle(w255) -> (w251:string[])
                n151 = Match First String(2:w251, 3:w256) -> (0:w252:i32)  [unwired: 1 out]
                n152 = property on="Test Ring" class="Ring (strict)"("Value"=w252, "Strings []"=w251) -> ()  [unwired: 2 in, 2 out]
                n153 = property on="Test Ring" class="Ring (strict)"("Visible"=TRUE) -> ()  [unwired: 2 in, 2 out]
                n154 = property on="Test Slider" class="Slide (strict)"("Visible"=FALSE) -> ()  [unwired: 2 in, 2 out]
              }
              frame "Exposure Priority  **" {
                n155 = Index Array(array=w263, index=3) -> (element=w264:cluster{string[]})
                n156 = call <vilib>:"NT Read String.vi"("Name"=w266) -> ("String"=w265:string)  [unwired: 9 in, 1 out]
                n157 = Unbundle(w264) -> (w260:string[])
                n158 = Match First String(2:w260, 3:w265) -> (0:w261:i32)  [unwired: 1 out]
                n159 = property on="Test Ring" class="Ring (strict)"("Value"=w261, "Strings []"=w260) -> ()  [unwired: 2 in, 2 out]
                n160 = property on="Test Ring" class="Ring (strict)"("Visible"=TRUE) -> ()  [unwired: 2 in, 2 out]
                n161 = property on="Test Slider" class="Slide (strict)"("Visible"=FALSE) -> ()  [unwired: 2 in, 2 out]
              }
              frame "Color Enable  **" {
                n162 = Index Array(array=w272, index=4) -> (element=w273:cluster{string[]})
                n163 = call <vilib>:"NT Read String.vi"("Name"=w275) -> ("String"=w274:string)  [unwired: 9 in, 1 out]
                n164 = Unbundle(w273) -> (w269:string[])
                n165 = Match First String(2:w269, 3:w274) -> (0:w270:i32)  [unwired: 1 out]
                n166 = property on="Test Ring" class="Ring (strict)"("Value"=w270, "Strings []"=w269) -> ()  [unwired: 2 in, 2 out]
                n167 = property on="Test Ring" class="Ring (strict)"("Visible"=TRUE) -> ()  [unwired: 2 in, 2 out]
                n168 = property on="Test Slider" class="Slide (strict)"("Visible"=FALSE) -> ()  [unwired: 2 in, 2 out]
              }
              frame Default {
                n169 = property on="Test Ring" class="Ring (strict)"("Visible"=FALSE) -> ()  [unwired: 2 in, 2 out]
                n170 = property on="Test Slider" class="Slide (strict)"("Visible"=FALSE) -> ()  [unwired: 2 in, 2 out]
              }
              frame "Brightness  **", "Color Level  **", "Compression  **", "FPS  **", "Sharpness  **" {
                n171 = call <vilib>:"NT Read Number.vi"("Name"=w281) -> ("Numeric"=w280:dbl)  [unwired: 9 in, 1 out]
                n172 = local write "Test Slider"(w280) -> ()
                n173 = property on="Test Slider" class="Slide (strict)"("Visible"=TRUE, "Scale.Maximum"=100.0 ("Scale.Range:Maximum")) -> ()  [unwired: 2 in, 2 out]
                n174 = property on="Test Ring" class="Ring (strict)"("Visible"=FALSE) -> ()  [unwired: 2 in, 2 out]
              }
            }
          }
        }
        n175 = property on="Progress" class="Clust (strict)"("Visible"=FALSE) -> ()  [unwired: 2 in, 2 out]
      }
      event "Test Name": Mouse Enter {
        # "Populate the ring with the list of tests"
        n176 = event-data() -> ()  [unwired: 1 in, 1 out]
        n177 = call <vilib>:"NT Read String Array.vi"("Name"="/TestMode/TestList") -> ("String Array"=w290:string[])  [unwired: 9 in, 1 out]
        n178 = Build Array (concatenate)("Select the test to run...", w290) -> (w289:string[])
        n179 = property on="Test Name" class="Ring (strict)"("Strings []"=w289) -> ()  [unwired: 2 in, 2 out]
      }
      event "Test Name": Value Change {
        w293 = FALSE ("Visible")
        # "Tell the robot the test name to run"
        n180 = event-data() -> ("NewVal"=w297:u16)  [unwired: 1 in]
        n181 = property on="Test Name" class="Ring (strict)"() -> ("Strings []"=w298:string[])  [unwired: 2 in, 2 out]
        n182 = local write "Progress"(T7 {"Test Progress"=0, "Test Progress Text"=""} ("Progress")) -> ()
        n183 = Index Array(array=w298, index=w297) -> (element=w296:string)
        n184 = call <vilib>:"NT Write String.vi"("String"=w296, "Name"="/TestMode/TestName") -> ()  [unwired: 9 in, 1 out]
        n185 = property on="Progress" class="Clust (strict)"("Visible"=TRUE) -> ()  [unwired: 2 in, 2 out]
        n186 = property on="Motor" class="Clust (strict)"("Visible"=w293) -> ()  [unwired: 2 in, 2 out]
        n187 = property on="Test Slider" class="Slide (strict)"("Visible"=w293) -> ()  [unwired: 2 in, 2 out]
        n188 = property on="On/Off" class="Bool (strict)"("Visible"=w293) -> ()  [unwired: 2 in, 2 out]
        n189 = property on="Rev/Fwd" class="Clust (strict)"("Visible"=w293) -> ()  [unwired: 2 in, 2 out]
        n190 = property on="Test Ring" class="Ring (strict)"("Visible"=w293) -> ()  [unwired: 2 in, 2 out]
      }
      event "Select Auto": Mouse Enter {
        # "Populate the combo box with the list of autonomous options"
        n191 = event-data() -> ()  [unwired: 1 in, 1 out]
        n192 = call <vilib>:"NT Read String Array.vi"("Name"="Auto List") -> ("String Array"=w300:string[])  [unwired: 9 in, 1 out]
        n193 = property on="Select Auto" class="CmbBox"("Strings[]"=w300) -> ()  [unwired: 2 in, 2 out]
      }
      event "Select Auto": Value Change {
        # "User modified the Auto Selection. Write to NT variable so robot knows."
        n194 = event-data() -> ("NewVal"=w304:string)  [unwired: 1 in]
        n195 = call <vilib>:"NT Write String.vi"("String"=w304, "Name"="Auto Selector") -> ()  [unwired: 9 in, 1 out]
      }
      event "Command Selection": Value Change {
        # "Get the params and show in table"
        n196 = event-data() -> ("NewVal"=w311:i32)  [unwired: 1 in]
        n197 = property on="Command Selection" class="MCListbox (strict)"() -> ("ItemNames"=w309:string[][])  [unwired: 2 in, 2 out]
        n198 = call <vilib>:"WPI_DashboardUpdate Command Params.vi"("NewVal"=w311, "Commands"=w309, "Param Tbl"=w310) -> ()  [unwired: 8 in, 1 out]
      }
      event "Execute Command": Value Change {
        # "Started one, Unique ID holds\nresponse"
        n199 = event-data() -> ()  [unwired: 1 in, 1 out]
        n200 = property on="Command Selection" class="MCListbox (strict)"() -> ("ItemNames"=w323:string[][])  [unwired: 2 in, 2 out]
        n201 = Index Array(array=w323, index (row)="Command Selection", index (col)=0) -> (element=w321:string)
        n202 = call <vilib>:"Invoke Commands.vi"("Command Params"="Command Params", "Function Name"=w321) -> ("Params"=w317:u8, "Started"=w316:bool)  [unwired: 7 in, 1 out]
        n203 = Array Subset(array="Command Params", length (row)=w317) -> (w318:string[][])  [unwired: 3 in]
        n204 = Select(t="Executing" ("Cmd Status"), s=w316, f="" ("Cmd Status")) -> (s? t:f=→"Cmd Status":string)
      }
      event "Command Selection": Double Click {
        n205 = event-data() -> ("Row"=w333:i32)  [unwired: 1 in]
        n206 = property on="Command Selection" class="MCListbox (strict)"() -> ("ItemNames"=w336:string[][])  [unwired: 2 in, 2 out]
        n207 = local read "Command Params"() -> (w331:string[][])
        n208 = Index Array(array=w336, index (row)=w333, index (col)=0) -> (element=w334:string)
        n209 = call <vilib>:"Invoke Commands.vi"("Command Params"=w331, "Function Name"=w334) -> ("Params"=w330:u8, "Started"=w325:bool)  [unwired: 7 in, 1 out]
        n210 = Array Subset(array=w331, length (row)=w330) -> (w329:string[][])  [unwired: 3 in]
        n211 = Select(t="Executing" ("Cmd Status"), s=w325, f="" ("Cmd Status")) -> (s? t:f=w326:string)
        n212 = local write "Cmd Status"(w326) -> ()
      }
      event "CheckList": Double Click {
        # "Shift clears all"
        # "Update symbols on the listbox"
        n213 = event-data() -> ("PlatMods.Shift"=w339:bool, "Row"=w341:i32)  [unwired: 1 in]
        n214 = case shown="True" w339 {
          tunnel: w341 -> [w345 _]
          tunnel: 1 -> [w344 _]
          frame False {
            n215 = property on="CheckList" class="LstBox (strict)"() -> ("Item Symbols"=w343:i32[])  [unwired: 2 in, 2 out]
            n216 = Replace Array Subset(array=w343, new element=w344, index=w345) -> (w342:i32[])
            n217 = property on="CheckList" class="LstBox (strict)"("Item Symbols"=w342) -> ()  [unwired: 2 in, 2 out]
          }
          frame True {
            w346 = 0 ("Top Row")
            n218 = property on="CheckList" class="LstBox (strict)"() -> ("Number of Rows"=w348:u32)  [unwired: 2 in, 2 out]
            n219 = Initialize Array(0, w348) -> (w347:i32[])
            n220 = property on="CheckList" class="LstBox (strict)"("Top Row"=w346, "Value"=w346, "Item Symbols"=w347) -> ()  [unwired: 2 in, 2 out]
          }
        }
      }
      event "CheckList": Key Down {
        # "Update symbols on the listbox\nLeft and right keys check and uncheck"
        n221 = event-data() -> ("VKey"=w353:T22)  [unwired: 1 in]
        n222 = case shown="\"Left\", \"Right\"" w353 {
          selector: w353 -> [w358 _]
          tunnel: eventvkey."Left" ("VKey") -> [w356 _]
          frame "Left", "Right" {
            n223 = Equal?(x=w356, y=w358) -> (x = y?=w357:bool)
            n224 = Select(t=0, s=w357, f=1) -> (s? t:f=w359:i32)
            n225 = property on="CheckList" class="LstBox (strict)"() -> ("Item Symbols"=w362:i32[])  [unwired: 2 in, 2 out]
            n226 = Replace Array Subset(array=w362, new element=w359, index="CheckList") -> (w361:i32[])
            n227 = property on="CheckList" class="LstBox (strict)"("Item Symbols"=w361) -> ()  [unwired: 2 in, 2 out]
          }
          frame Default {
          }
        }
      }
      event "DB Camera Config": Value Change {
        # "Show or hide the cluster of controls, store in ini file"
        n228 = event-data() -> ("NewVal"=w367:bool)  [unwired: 1 in]
        n229 = case shown="False" w367 {
          tunnel: w366 -> [w376 _]
          tunnel: [w369 w387] -> w365
          tunnel: w364 -> [w368 w387]
          frame False {
            w383 = "Camera"
            w386 = FALSE ("Visible")
            n230 = local read "Camera Settings"() -> (w375:T1)
            n231 = Index Array(array=w376) -> (element=w379:cluster{string[]})  [unwired: 1 in]
            n232 = Unbundle(w375) -> ("Frame Rate"=w374:i32, "Compression"=w373:i32, "Size"=w377:u16)
            n233 = Unbundle(w379) -> (w378:string[])
            n234 = Index Array(array=w378, index=w377) -> (element=w372:string)
            n235 = call-poly <vilib>:"Write Key.vi"("section"=w383, "value"=w372, "key"="Size", "refnum"=w368) -> ("refnum out"=w385:T20)  [unwired: 2 in, 5 out]
            n236 = call-poly <vilib>:"Write Key.vi"("section"=w383, "value"=w374, "key"="FrameRate", "refnum"=w385) -> ("refnum out"=w384:T20)  [unwired: 1 in, 6 out]
            n237 = property on="Camera Settings" class="Clust (strict)"("Visible"=w386) -> ()  [unwired: 2 in, 2 out]
            n238 = local write "DB Camera Config"(w386) -> ()
            n239 = call-poly <vilib>:"Write Key.vi"("section"=w383, "value"=w373, "key"="Compression", "refnum"=w384) -> ("refnum out"=w370:T20)  [unwired: 1 in, 6 out]
            n240 = call <vilib>:"Close Config Data.vi"("refnum"=w370) -> ("file path"=w371:path)  [unwired: 2 in, 8 out]
            n241 = call <vilib>:"Open Config Data.vi"("configuration file path"=w371) -> ("refnum"=w369:T20)  [unwired: 8 in, 2 out]
          }
          frame True {
            n242 = property on="Camera Settings" class="Clust (strict)"("Visible"=TRUE) -> ()  [unwired: 2 in, 2 out]
          }
        }
      }
      event "Camera Settings": Value Change {
        # "Update summary string when any elements of DB camera change"
        n243 = event-data() -> ("NewVal"=w401:T1)  [unwired: 1 in]
        n244 = Index Array(array=w397) -> (element=w396:cluster{string[]})  [unwired: 1 in]
        n245 = Unbundle(w401) -> ("Frame Rate"=w392:i32, "Compression"=w391:i32, "Size"=w394:u16)
        n246 = Unbundle(w396) -> (w395:string[])
        n247 = Index Array(array=w395, index=w394) -> (element=w393:string)
        n248 = Format Into String(format string="%s   %dfps   %d%%", w393, w392, w391) -> (resulting string=w398:string)  [unwired: 2 in, 1 out]
        n249 = Build Array(w398) -> (w399:string[])
        n250 = property on="DB Camera Config" class="Bool (strict)"("Strings [4]"=w399) -> ()  [unwired: 2 in, 2 out]
      }
      event "Motor.Enable": Value Change {
        # "When the test mode otor enable helper is set, update that\ntree row item's value"
        n251 = event-data() -> ("NewVal"=w408:bool)  [unwired: 1 in]
        n252 = Unbundle("Motor") -> ("Value"=w407:dbl)  [unwired: 1 out]
        n253 = Select(t=w407, s=w408, f=0.0) -> (s? t:f=w405:dbl)
        n254 = call <vilib>:"NT Write Number.vi"("Numeric"=w405, "Name"=w404) -> ()  [unwired: 9 in, 1 out]
      }
      event "Test Slider": Value Change {
        # "When the test mode slider helper is set, update that\ntree row item's value"
        n255 = event-data() -> ("NewVal"=w412:dbl)  [unwired: 1 in]
        n256 = call <vilib>:"NT Write Number.vi"("Numeric"=w412, "Name"=w413) -> ()  [unwired: 9 in, 1 out]
      }
      event "On/Off": Value Change {
        # "When the test mode on/off helper value is set, update that\ntree row item's value"
        n257 = event-data() -> ("NewVal"=w418:bool)  [unwired: 1 in]
        n258 = Boolean To (0,1)(Boolean=w418) -> (0, 1=w417:i16)
        n259 = call <vilib>:"NT Write Number.vi"("Numeric"=w417, "Name"=w416) -> ()  [unwired: 9 in, 1 out]
      }
      event "Rev/Fwd": Value Change {
        # "When the test mode helper value for relays is set, update that\ntree row item's value"
        n260 = event-data() -> ("NewVal.Forward"=w427:bool, "NewVal.Reverse"=w426:bool)  [unwired: 1 in]
        n261 = Boolean To (0,1)(Boolean=w427) -> (0, 1=w423:i16)
        n262 = Boolean To (0,1)(Boolean=w426) -> (0, 1=w425:i16)
        n263 = Negate(x=w425) -> (-x=w424:i16)
        n264 = Add(x=w423, y=w424) -> (x+y=w422:i16)
        n265 = call <vilib>:"NT Write Number.vi"("Numeric"=w422, "Name"=w421) -> ()  [unwired: 9 in, 1 out]
      }
      event "Test Ring": Value Change {
        # "When a test mode helper value is selected from the ring,\nset the tree item's variable to the string value"
        n266 = event-data() -> ("NewVal"=w432:u16)  [unwired: 1 in]
        n267 = property on="Test Ring" class="Ring (strict)"() -> ("Strings []"=w433:string[])  [unwired: 2 in, 2 out]
        n268 = Index Array(array=w433, index=w432) -> (element=w431:string)
        n269 = call <vilib>:"NT Write String.vi"("String"=w431, "Name"=w430) -> ()  [unwired: 9 in, 1 out]
      }
      event "Rec Mode": Value Change {
        # "Update globals for recording mode and path to read log from.\nClear when logging and let NetworkTables set path for vision to\nuse."
        n270 = event-data() -> ("NewVal"=w445:enum32{"Stop", "Record", "Playback"})  [unwired: 1 in]
        n271 = global write "WPI_DashboardLogging Global.vi" "Logging Filename"(path "") -> ()
        n272 = global write "WPI_DashboardLogging Global.vi" "Recording"(w445) -> ()
        n273 = case shown="\"Playback\"" w445 {
          tunnel: w444 -> [_ w447 w456]
          tunnel: [_ _ w455] -> w441
          tunnel: [_ _ w454] -> _
          tunnel: w439 -> [_ _ w452]
          tunnel: cluster{i32, i32} {-250, 170} -> [_ _ w451]
          tunnel: [_ _ T23 {"Image Size"=TRUE, "Image Type"=TRUE, "Pixel Value"=TRUE, "ROI Information"=TRUE, "Zoom Factor"=FALSE} ("Image Information Shown:All Elements")] -> w437
          tunnel: [_ _ TRUE ("Zoom Factor")] -> w436
          tunnel: w435 -> [_ _ w448]
          frame Default {
          }
          frame "Stop", "Record" {
            # "Place Window too"
            n274 = invoke class="VI" method="FP.Close"(reference=w447) -> (reference out=w446:refnum<vi>)  [unwired: 2 in, 2 out]
            n275 = invoke class="VI" method="Abort VI"(reference=w446) -> ()  [unwired: 2 in, 3 out]
          }
          frame "Playback" {
            n276 = call "Open Playback Panel.vi"("Offset"=w451, "DB VI Ref"=w452, "Playback in"=w456) -> ("Playback out"=w453:refnum<vi>)  [unwired: 8 in]
            n277 = register-events(w453, w448) -> (reference out=w455:refnum<event-registration>, error out=w454:errorcluster)  [unwired: 2 in]
          }
        }
        n278 = property on="Camera Image" class="ImageControl"("Image Information Shown"=w437, "Image Information Visible"=w436) -> ()  [unwired: 2 in, 2 out]
        n279 = call <vilib>:"WPI_DashboardNT Log FieldName Cache.vi"("Operation"=enum16{"Lookup/Add", "Index", "Clear"}."Clear") -> ()  [unwired: 8 in, 3 out]
      }
      event Panel Close {
        w458 = enum32{"Stop", "Record", "Playback"}."Stop" ("Rec Mode")
        # "Playback window has been closed, abort"
        n280 = event-data() -> ()  [unwired: 1 in, 4 out]
        n281 = local write "Rec Mode"(w458) -> ()
        n282 = global write "WPI_DashboardLogging Global.vi" "Recording"(w458) -> ()
      }
      event Panel Close {
        # "Abort playback window and ourself"
        n283 = event-data() -> ()  [unwired: 1 in, 4 out]
        n284 = invoke class="VI" method="FP.Close"(reference=w464) -> (reference out=w463:refnum<vi>)  [unwired: 2 in, 2 out]
        n285 = invoke class="VI" method="Abort VI"(reference=w463) -> (error out=w462:errorcluster)  [unwired: 2 in, 2 out]
        n286 = invoke class="VI" method="Abort VI"(error in=w462) -> ()  [unwired: 2 in, 3 out]
      }
      event User Event {
        n287 = event-data() -> ("IDs"=w472:cluster{"RPC field ID":u16, "Unique ID":u16}, "String"=w471:string)  [unwired: 1 in]
        n288 = Bundle("IDs"=w472, "String"=w471) -> (w470:T10)  [unwired: 1 in]
        n289 = call <vilib>:"Retrieve RPC Response.vi"("RPC Response"=w470) -> ("Output"=w467:string[][])  [unwired: 10 in]
        n290 = Build Array (concatenate)(w465, w467) -> (w466:string[][])
        n291 = local write "Command Params"(w466) -> ()
        n292 = local write "Cmd Status"("" ("Cmd Status")) -> ()
      }
      event "Vision": Value Change {
        # "Enable/Disable Compression slider.\nHW USB is hard-coded into the camera"
        n293 = event-data() -> ("NewVal"=w479:u16)  [unwired: 1 in]
        n294 = Equal?(x=w479, y=u32 2 ("milliseconds to wait")) -> (x = y?=w477:bool)
        n295 = Select(t=T24."Disabled and Grayed Out" ("Disabled"), s=w477, f=T24."Enabled" ("Disabled")) -> (s? t:f=w474:T24)
        n296 = property on="Compression" class="Slide (strict)"("DisabledEnum"=w474) -> ()  [unwired: 2 in, 2 out]
      }
      event "Tree": Double Click {
        n297 = event-data() -> ("PlatMods"=w484:T27, "Tag"=w483:string)  [unwired: 1 in]
        n298 = Unbundle(w484) -> ("Shift"=w482:bool)  [unwired: 4 out]
        n299 = Not(x=w482) -> (.not. x?=w481:bool)
        n300 = call <vilib>:"NT Update Persistence.vi"("Persistence"=w481, "Name"=w483) -> ()  [unwired: 9 in, 1 out]
      }
    }
  }
  n301 = while {
    tunnel: w50 -> [w488]
    i -> [w491]
    stop <- FALSE stop-if-true
    n302 = Wait (ms)(milliseconds to wait=u32 100) -> ()  [unwired: 1 out]
    n303 = case shown="\"Playback\"" "Rec Mode" {
      tunnel: w491 -> [_ _ w506]
      tunnel: [u32 2829099 ("Base Color") u32 11141120 ("Target Color") w495] -> w487
      frame "Stop", Default {
        # "Reset the color, extra updates don't cost much"
      }
      frame "Record" {
      }
      frame "Playback" {
        # "Playback"
        n304 = Quotient & Remainder(x=w506, y=u32 50 ("milliseconds to wait")) -> (x-y*floor(x/y)=w502:u32)  [unwired: 1 out]
        n305 = Divide(x=w502, y=u32 50 ("milliseconds to wait")) -> (x/y=w499:dbl)
        n306 = Multiply(x=6.283185307179586, y=w499) -> (x*y=w504:dbl)
        n307 = Sine(x=w504) -> (sin(x)=w503:dbl)
        n308 = Absolute Value(x=w503) -> (abs(x)=w496:dbl)
        n309 = call "Interpolate RGB Color.vi"("Proportion"=w496, "Target Color"=u32 30976, "Base Color"=u32 2829099) -> ("Result Color"=w495:u32)  [unwired: 8 in]
      }
    }
    n310 = property class="Pane"(reference=w488, "PaneColor"=w487) -> ()  [unwired: 1 in, 2 out]
  }
  n311 = local write "Dashboard Tab"(T2."Drive" ("Dashboard Tab")) -> ()
  n312 = property on="On/Off" class="Bool (strict)"("Visible"=w18) -> ()  [unwired: 2 in, 2 out]
  n313 = property on="Motor" class="Clust (strict)"("Visible"=w18) -> ()  [unwired: 2 in, 2 out]
  n314 = property on="Progress" class="Clust (strict)"("Visible"=w18) -> ()  [unwired: 2 in, 2 out]
  n315 = property on="Test Ring" class="Ring (strict)"("Visible"=w18) -> ()  [unwired: 2 in, 2 out]
  n316 = property on="Rev/Fwd" class="Clust (strict)"("Visible"=w18) -> ()  [unwired: 2 in, 2 out]
  n317 = property on="Camera Settings" class="Clust (strict)"("Visible"=w18) -> ()  [unwired: 2 in, 2 out]
  n318 = while {
    tunnel: u16 1741 ("timeout ms (25000)") -> [w508]
    stop <- FALSE stop-if-true
    n319 = TCP Create Listener(10:w508) -> (0:w507:errorcluster, 3:w509:refnum<k5>)  [unwired: 4 in, 1 out]
    n320 = case shown="No Error" w507 {
      selector: w507 -> [w511 _]
      tunnel: w509 -> [w512 _]
      frame No Error {
        n321 = while {
          tunnel: w512 -> [w515]
          tunnel: w511 -> [w514]
          stop <- FALSE stop-if-true
          n322 = TCP Wait On Listener(8:w514, 11:w515) -> (0:w516:errorcluster, 4:w517:refnum<k5>)  [unwired: 2 in, 3 out]
          n323 = local write "TCP"(w517) -> ()
          n324 = case shown="No Error" w516 {
            frame No Error {
            }
            frame Error {
              n325 = Wait (ms)(milliseconds to wait=u32 1000) -> ()  [unwired: 1 out]
            }
          }
        }
      }
      frame Error {
        n326 = Wait (ms)(milliseconds to wait=u32 1000) -> ()  [unwired: 1 out]
      }
    }
  }
  n327 = local write "DB Camera Config"(w18) -> ()
  n328 = local write "Command Params"(string[][] [] ("Command Params")) -> ()
  n329 = global write "WPI_DashboardLogging Global.vi" "Recording"(w44) -> ()
  n330 = local write "Command Selection"(u16 0 ("milliseconds to wait")) -> ()
  n331 = local write "Rec Mode"(w44) -> ()
  n332 = call "IMAQ Create"("Image Name"="Dashboard Image 2", "Image Type"=w2) -> ("New Image"=w1:T8)  [unwired: 2 in, 2 out]
  n333 = while {
    tunnel: w62 -> [w530]
    tunnel: w61 -> [_]
    tunnel: [w531] -> _
    tunnel: w1 -> [w521]
    i -> [w531]
    stop <- FALSE stop-if-true
    # "Optionally read the DB image,\nlog, or retrieve images from a\nlogged match"
    n334 = local read "Rec Mode"() -> (w525:enum32{"Stop", "Record", "Playback"})
    n335 = local read "Camera IP"() -> (w523:string)
    n336 = call "836_MultiCameraRead MJPG for Dashboard.vi"("Camera Settings"="Camera Settings", "port"=u16 1180, "Rec Mode"=w525, "Camera IP"=w523, "Camera Mode"="Vision", "Refnum in"=w530) -> ("Active"=w528:bool, "Refnum out"=w529:T8, "FPS"=w527:dbl, "Bandwidth (Mbps)"=w522:dbl)  [unwired: 2 in]
    "Mbps" <- w522
    n337 = case shown="True" w528 {
      tunnel: w529 -> [_ w542]
      tunnel: w522 -> [_ w541]
      tunnel: w527 -> [_ w540]
      tunnel: w521 -> [_ w538]
      frame False {
        w533 = u32 1985280 ("Color Box")
        # "Sleep for 500ms"
        n338 = Bundle("Color Box"=w533, "Color Box"=w533) -> (w535:cluster{"Color Box":u32, "Color Box":u32})  [unwired: 1 out]
        n339 = Build Array(w535) -> (w534:cluster{"Color Box":u32, "Color Box":u32}[])
        n340 = property on="Mbps LED" class="Bool (strict)"("Colors [4]"=w534) -> ()  [unwired: 2 in, 2 out]
        n341 = Wait Until Next ms Multiple(millisecond multiple=u32 500) -> ()  [unwired: 1 out]
      }
      frame True {
        # "Here is where you would annotate,\npossibly process, and display the image"
        # "Update Mbps LED"
        n342 = call "IMAQ Clear Overlay"("Image"=w542) -> ("error out"=w546:errorcluster, "Image Out"=w537:T8)  [unwired: 2 in, 7 out]
        n343 = case shown="Default" w541 {
          tunnel: [u32 6618880 ("Color Box") u32 16776722 ("Color Box") u32 16716800 ("Color Box")] -> w543
          frame Default {
          }
          frame 4, 5 {
          }
          frame 6.. {
          }
        }
        n344 = Unbundle By Name(w546) -> ("status"=w547:bool)
        n345 = Bundle("Color Box"=w543, "Color Box"=w543) -> (w545:cluster{"Color Box":u32, "Color Box":u32})  [unwired: 1 out]
        n346 = property on="Image Message" class="Str"("Visible"=w547) -> ()  [unwired: 2 in, 2 out]
        n347 = Build Array(w545) -> (w544:cluster{"Color Box":u32, "Color Box":u32}[])
        n348 = property on="Mbps LED" class="Bool (strict)"("Colors [4]"=w544) -> ()  [unwired: 2 in, 2 out]
        n349 = call "IMAQ ImageToImage 2"("Image Dst"=w537, "Image Src (Small)"=w538, "Image Src (Large)"=w537) -> ("Image Dst Out"=→"Camera Image":T8)  [unwired: 7 in, 1 out]
        "fps" <- w540
      }
    }
  }
  n350 = while {
    tunnel: w1 -> [w560]
    tunnel: [w561] -> _
    i -> [w561]
    stop <- FALSE stop-if-true
    # "Optionally read the DB image,\nlog, or retrieve images from a\nlogged match"
    n351 = local read "Rec Mode"() -> (w555:enum32{"Stop", "Record", "Playback"})
    n352 = local read "Camera IP"() -> (w553:string)
    n353 = call "836_MultiCameraRead MJPG for Dashboard.vi"("Camera Settings"="Camera Settings 2", "port"=u16 1181, "Rec Mode"=w555, "Camera IP"=w553, "Camera Mode"="Vision 2", "Refnum in"=w560) -> ("Active"=w558:bool, "Refnum out"=w559:T8, "FPS"=w557:dbl, "Bandwidth (Mbps)"=w552:dbl)  [unwired: 2 in]
    "Mbps 2" <- w552
    n354 = case shown="True" w558 {
      tunnel: w559 -> [_ w569]
      tunnel: w552 -> [_ w568]
      tunnel: w557 -> [_ w567]
      frame False {
        w563 = u32 1985280 ("Color Box")
        # "Sleep for 500ms"
        n355 = Bundle("Color Box"=w563, "Color Box"=w563) -> (w565:cluster{"Color Box":u32, "Color Box":u32})  [unwired: 1 out]
        n356 = Build Array(w565) -> (w564:cluster{"Color Box":u32, "Color Box":u32}[])
        n357 = property on="Mbps LED" class="Bool (strict)"("Colors [4]"=w564) -> ()  [unwired: 2 in, 2 out]
        n358 = Wait Until Next ms Multiple(millisecond multiple=u32 500) -> ()  [unwired: 1 out]
      }
      frame True {
        # "Here is where you would annotate,\npossibly process, and display the image"
        # "Update Mbps LED"
        n359 = call "IMAQ Clear Overlay"("Image"=w569) -> ("error out"=w573:errorcluster)  [unwired: 2 in, 8 out]
        n360 = case shown="Default" w568 {
          tunnel: [u32 6618880 ("Color Box") u32 16776722 ("Color Box") u32 16716800 ("Color Box")] -> w570
          frame Default {
          }
          frame 4, 5 {
          }
          frame 6.. {
          }
        }
        n361 = Unbundle By Name(w573) -> ("status"=w574:bool)
        n362 = Bundle("Color Box"=w570, "Color Box"=w570) -> (w572:cluster{"Color Box":u32, "Color Box":u32})  [unwired: 1 out]
        n363 = property on="Image Message" class="Str"("Visible"=w574) -> ()  [unwired: 2 in, 2 out]
        n364 = Build Array(w572) -> (w571:cluster{"Color Box":u32, "Color Box":u32}[])
        n365 = property on="Mbps LED" class="Bool (strict)"("Colors [4]"=w571) -> ()  [unwired: 2 in, 2 out]
        "fps 2" <- w567
      }
    }
  }
